vi "Move bimorph.vi"() -> ()   [LabVIEW 2010]
uses:
  <vilib>/express/express analysis/Spectral/XNode/ExpressSpectralMeasurementsBlockNode.xnode
  <vilib>/DAQmx/read.llb/DAQmx Read (Analog 2D DBL NChan NSamp).vi
  <vilib>/daqmx/miscellaneous.llb/DAQmx Fill In Error Info.vi
  <vilib>/express/express analysis/Spectral/Block/exnSpectralBlock spectral measurements peak poly.vi
  <vilib>/express/express analysis/Spectral/Block/exnSpectralBlock spectral measurements peak array WFM.vi
panel:
  out "Amplitude 2 (microns)":sgl=3.0 format="%.4f"
  in  "Load config file":bool
  out "Config file path":path
  in  "Save config file":bool
  in  "Axis":T1(radio)=enum."Radio Selection 3"
  in  "Bimorph scaling factor (?/V)":dbl=1.0
  out "FFT":cluster{"f0":dbl, "df":dbl, "magnitude":dbl[]}[](graph)
  out "Period (s)":dbl
  in  "Timing":T2={"Delay 1 (s)"=10.0, "Duration (s)"=10.0, "Delay 2 (s)"=10.0} {"Delay 2 (s)" step=0.5 format="%.1g"; "Duration (s)" step=0.5 format="%.1g"; "Delay 1 (s)" step=0.5 format="%.1g"}
  out "Coordinates":T3 {"Zcoordinate" format="%.4f"; "Ycoordinate" format="%.4f"; "Xcoordinate" format="%.4f"}
  out "Coordinates (microns)":T4={"Xcoordinate (microns)"=8589, "Ycoordinate (microns)"=6028, "Zcoordinate (microns)"=4319}
  out "Error":bool
  in  "Get start position":bool
  in  "Amplitude 0 (microns)":dbl format="%.4g"
  in  "Shell?":bool
  out "Amplitude index":i32=1
  out "File path":path caption="Saved file path"
  in  "Comments":string
  in  "Save?":bool=TRUE
  in  "stop":bool
  in  "Amplitudes":T5={"# of amplitudes"=1, "Amplitude type?"=0, "Amplitude 1 (microns)"=3.0, "Step size (microns)"=0.0, "Amplitude array (microns)"=[]} {"Amplitude array (microns)" format="%.4g"; "Step size (microns)" step=0.0625 format="%.4f"; "Amplitude 1 (microns)" format="%.4f"; "Amplitude type?" items=["Linear", "Array"]}
  in  "Sample rate (Hz)":dbl=2000.0 format="%.2f"
  out "WAITING?":bool
  in  "CONTINUE":bool
  in  "Switch":u8(slide) step=1 scale=0.0..2.0
  out "Bimorph voltage":cluster{dbl, dbl, "data":dbl[]}(graph)
  in  "AI max value":dbl=10.0 caption="Input Maximum Value" format="%0.2f"
  in  "AI min value":dbl=-10.0 caption="Input Minimum Value" format="%0.2f"
  in  "AI channels":tag="Dev2/ai0" caption="Input Physical Channel"
  # "Channel Parameters"
  # "STOP VI"
  # "IDLE"
  # "RUN"
  # "ai0: Bimorph signal from amplifier"
  # "ENTER BEFORE RUN."
  # "DECIDE BEFORE RUN."
  # "Log file key:\nFile name\nComments\nSample rate (Hz)\nDelay 1 (s)\nDuration (s)\nDelay 2 (s)\nX coordinate (microns)\nY coordinate (microns)\nZ coordinate (microns)\nBimorph scaling factor\nAmplitude 0 (microns)\n# of amplitudes\nAmplitude type (0=linear, 1=array)\nAmplitude 1 (microns)\nStep size (microns)\nSize of amplitude array\nAmpiltude array (microns)"
  # "Instructions:\n1. Run vi.\n2. In IDLE mode, specify the sample rate, the timing parameters, the bimorph scaling factor, and comments.\n3. Choose which axis to control, then get the start position (the baseline of the pulse), amplitude 0.\n4. Specify the amplitude parameters. Note that all amplitudes are absolute, not relative.\n5. Run the Shell if needed, and decide if you want to save.\n6. Click RUN.\n\nNotes:\n-The communication with the Sutter manipulator sometimes has errors. Try to visually confirm on the \nROE that the commanded move is what you want.\n-When setting the timing parameters, make sure to account for the time it takes for the manipulator to\nmove.\n-The minimum step size is 62.5 nm.\n\n-"
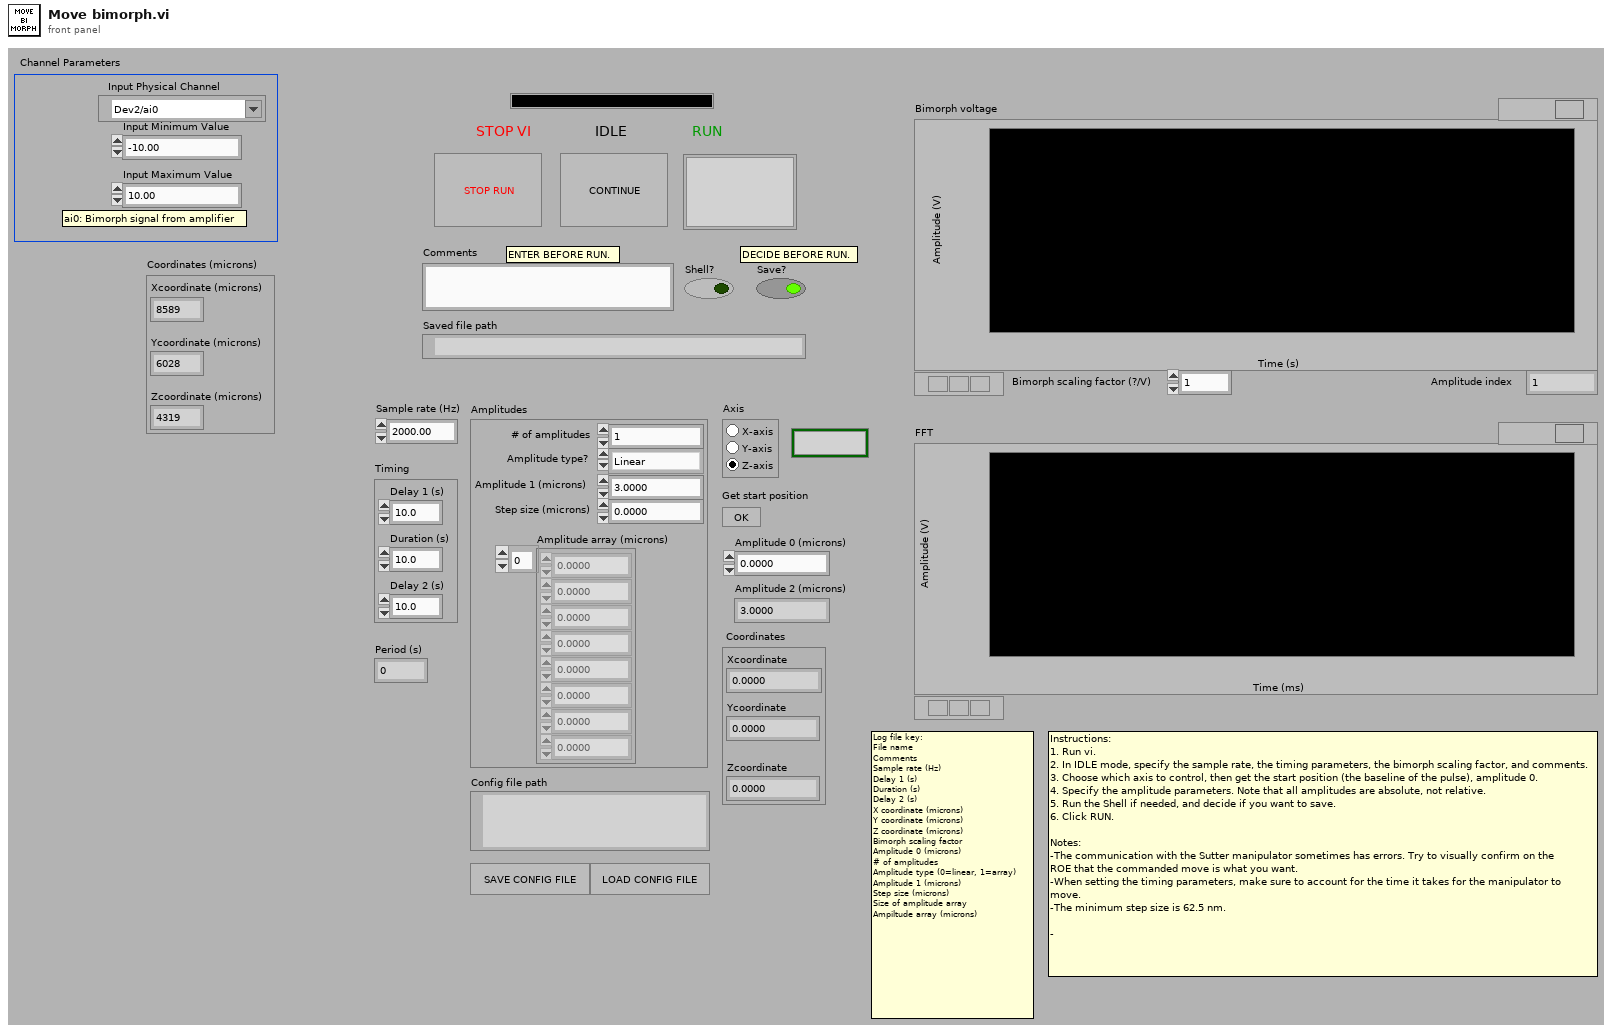
[diagram p1: front panel]
types:
  T1 = enum32{"Radio Selection 1", "Radio Selection 2", "Radio Selection 3"}
  T2 = cluster{"Delay 1 (s)":dbl, "Duration (s)":dbl, "Delay 2 (s)":dbl}
  T3 = cluster{"Xcoordinate ":dbl, "Ycoordinate":dbl, "Zcoordinate":dbl}
  T4 = cluster{"Xcoordinate (microns)":i32, "Ycoordinate (microns)":i32, "Zcoordinate (microns)":i32}
  T5 = cluster{"# of amplitudes":i32, "Amplitude type?":u16, "Amplitude 1 (microns)":sgl, "Step size (microns)":sgl, "Amplitude array (microns)":dbl[]}
  T6 = cluster{"name":string, "type desc":i16[], "flat data":string}[]
  T7 = cluster{"averaging mode":u16, "weighting mode":u16, "number of averages":u32}
  T8 = cluster{"dB On (F)":bool, "unwrap phase (F)":bool, "convert to degree (F)":bool}
  T9 = cluster{"Xcoordinate (not rounded)":dbl, "Ycoordinate (not rounded)":dbl, "Zcoordinate (not rounded)":dbl}
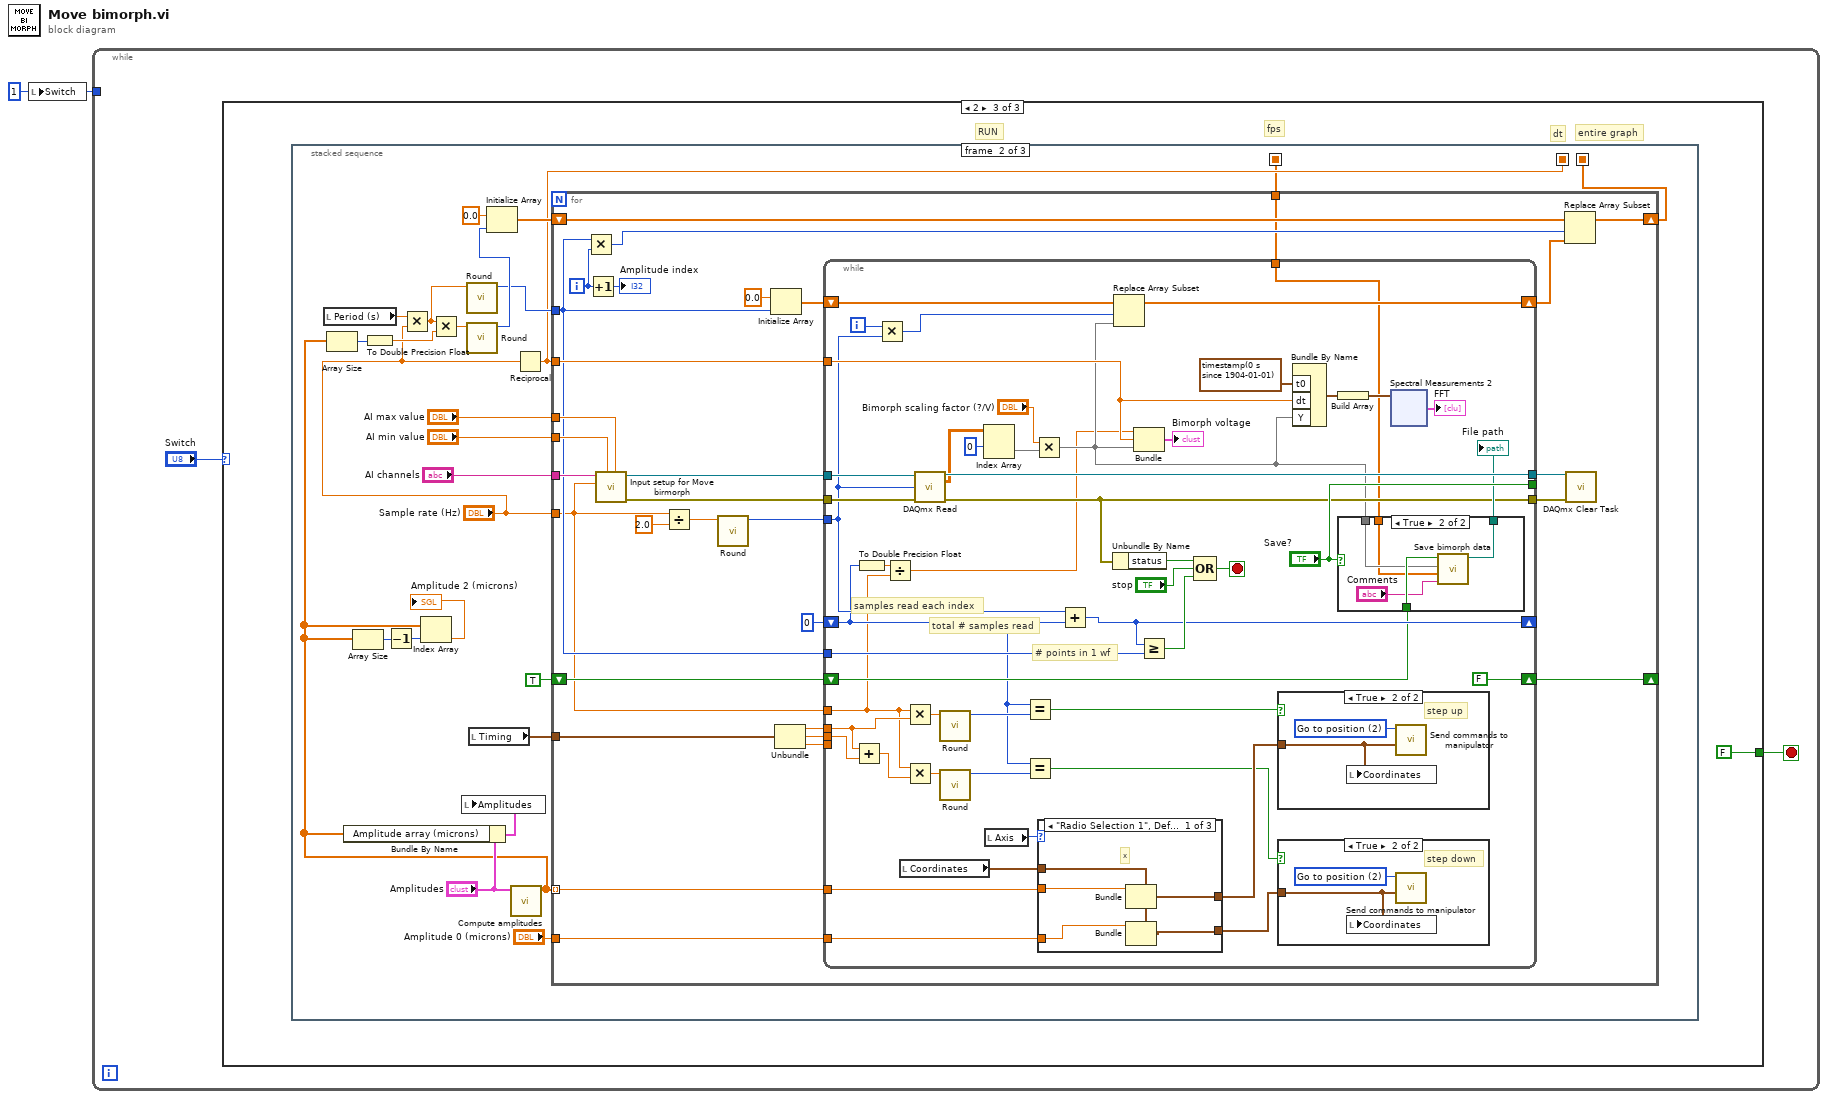
[diagram p0: block diagram]
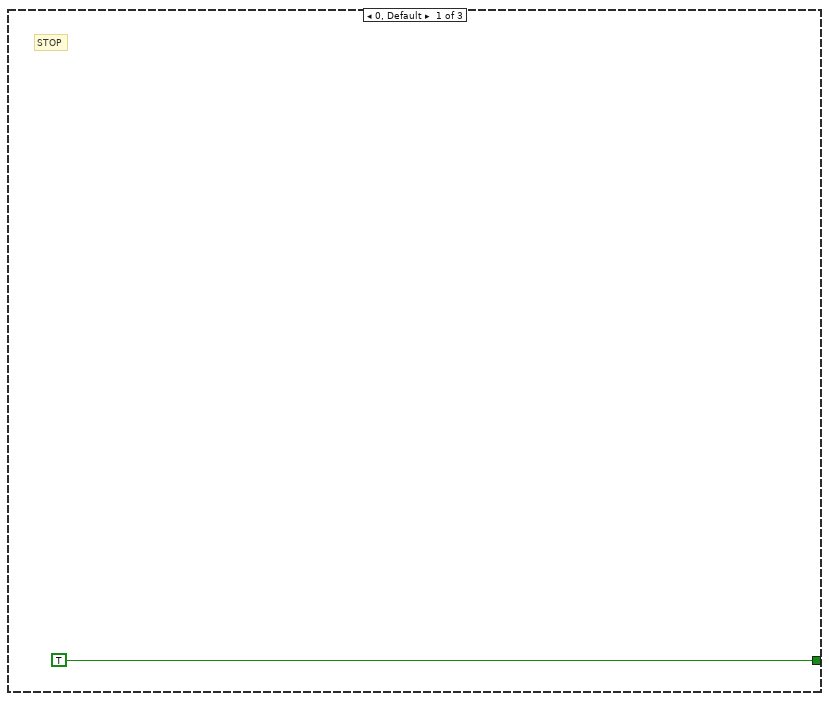
[diagram p2: hidden frame]
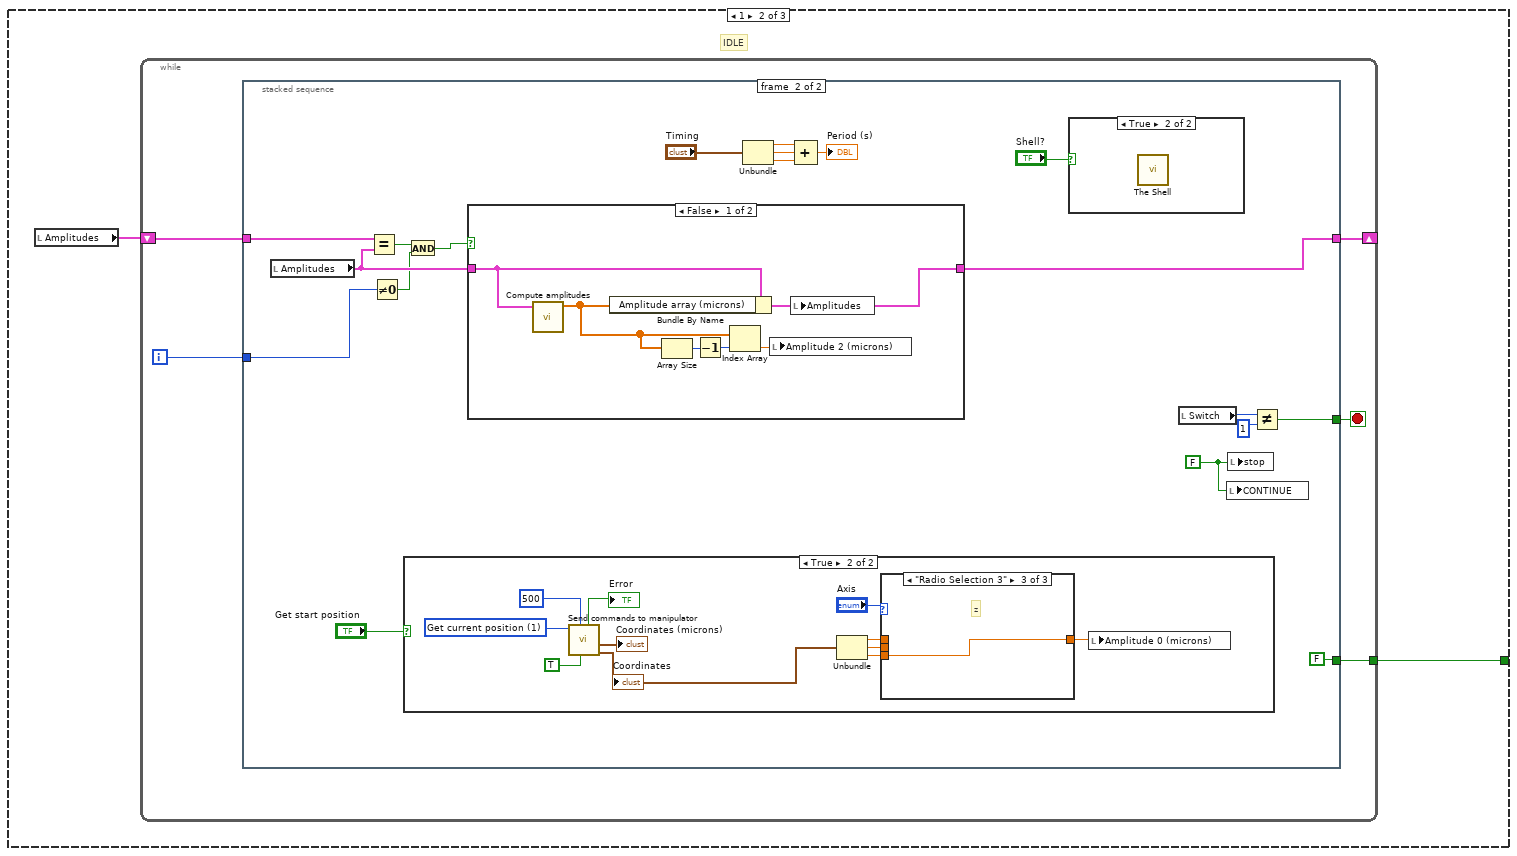
[diagram p3: hidden frame]
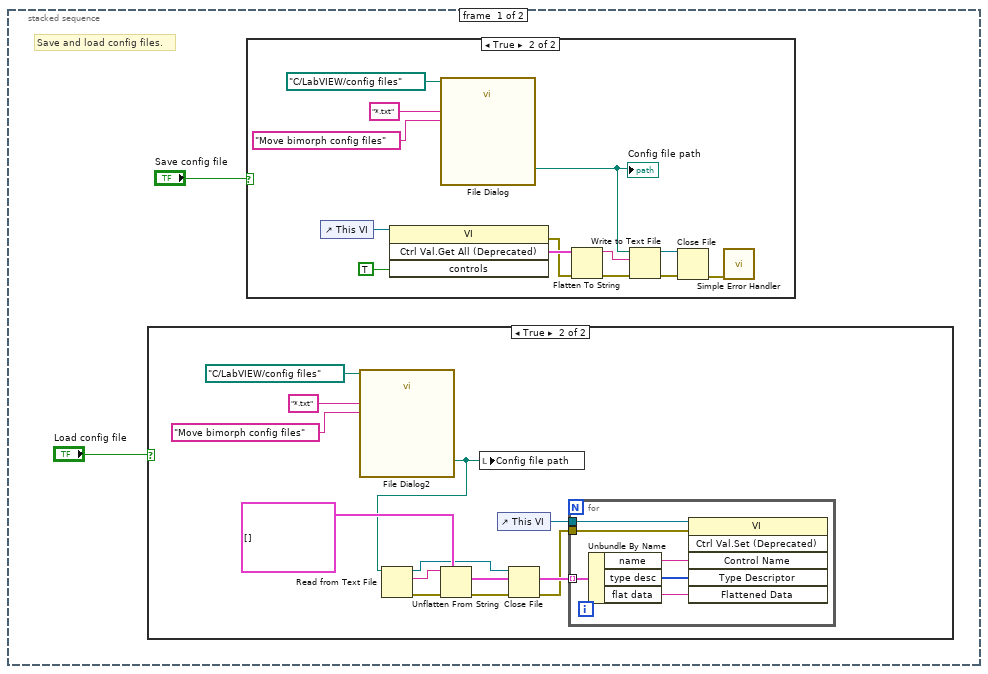
[diagram p4: hidden frame]
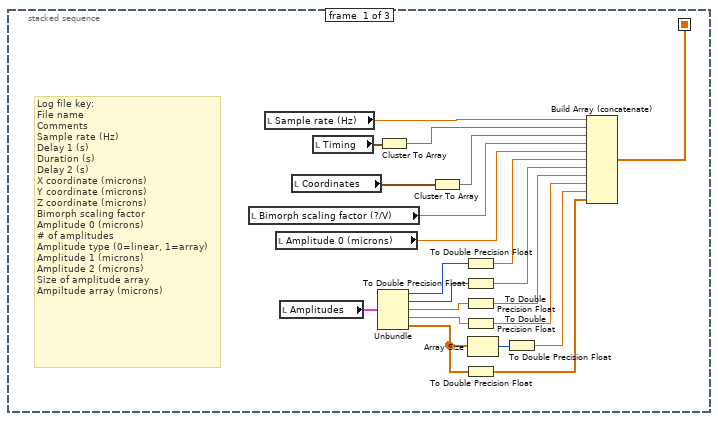
[diagram p12: hidden frame]
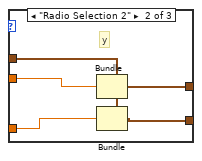
[diagram p14: hidden frame]
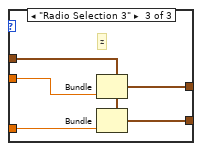
[diagram p15: hidden frame]
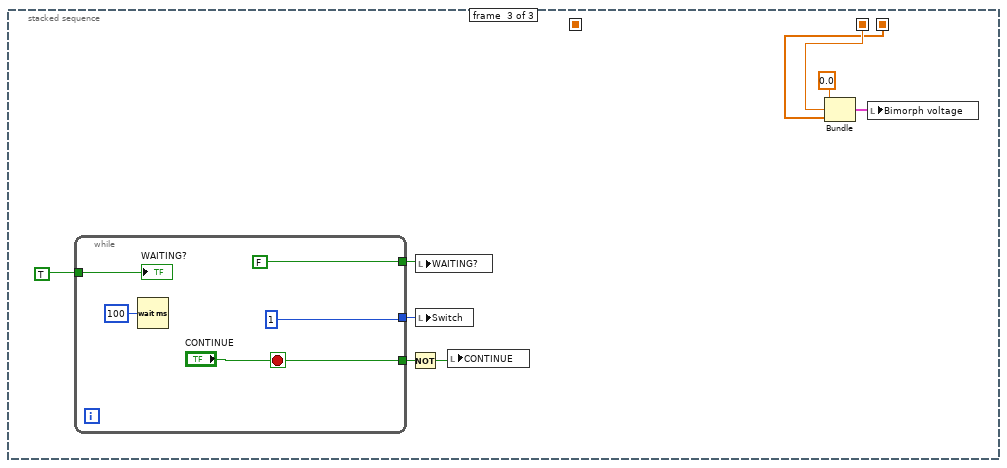
[diagram p18: hidden frame]
diagram:
  w1 = u8 1 ("Switch")
  n1 = local write "Switch"(w1) -> ()
  n2 = while {
    tunnel: w1 -> [_]
    stop <- w2 stop-if-true
    n3 = case shown="2" "Switch" {
      tunnel: [TRUE w6 FALSE] -> w2
      frame 0, Default {
        # "STOP"
      }
      frame 1 {
        # "IDLE"
        n4 = local read "Amplitudes"() -> (w5:T5)
        n5 = while {
          tunnel: [w9] -> w6
          shift-right: [w7] -> _
          shift-left: w5 -> [w8]
          i -> [w11]
          stop <- w10 stop-if-true
          n6 = stacked-sequence {
            tunnel: w11 -> [_ w47]
            tunnel: [_ w59] -> w10
            tunnel: [_ FALSE] -> w9
            tunnel: w8 -> [_ w51]
            tunnel: [_ w49] -> w7
            frame #0 {
              # "Save and load config files."
              n7 = case shown="True" "Load config file" {
                frame False {
                }
                frame True {
                  n8 = call "File Dialog2"("start path"=path "C:/LabVIEW/config files", "pattern (all files)"="*.txt", "pattern label"="Move bimorph config files") -> ("selected path"=w15:path)  [unwired: 9 in, 3 out]
                  n9 = Read from Text File(file (use dialog)=w15) -> (refnum out=w20:refnum<file>, text=w22:string, error out=w21:errorcluster)  [unwired: 1 in, 3 out]
                  n10 = Unflatten From String(type=T6 [] ("Control Value:Get All [Flattened]"), binary string=w22, error in (no error)=w21) -> (value=w24:T6, error out=w19:errorcluster)  [unwired: 3 out]
                  n11 = local write "Config file path"(w15) -> ()
                  n12 = control-ref of="This VI"() -> (w25:refnum<vi>)
                  n13 = Close File(refnum=w20, error in=w19) -> (error out=w14:errorcluster)  [unwired: 1 out]
                  n14 = for {
                    tunnel: w25 -> [w31]
                    tunnel: w24 -> [w30] mode=indexing
                    tunnel: w14 -> [w26]
                    n15 = Unbundle By Name(w30) -> ("name"=w29:string, "type desc"=w28:i16[], "flat data"=w27:string)
                    n16 = invoke class="VI" method="Ctrl Val.Set (Deprecated)"(reference=w31, error in=w26, "Control Name"=w29, "Type Descriptor"=w28, "Flattened Data"=w27) -> ()  [unwired: 1 in, 6 out]
                  }
                }
              }
              n17 = case shown="True" "Save config file" {
                frame False {
                }
                frame True {
                  n18 = control-ref of="This VI"() -> (w40:refnum<vi>)
                  n19 = invoke class="VI" method="Ctrl Val.Get All (Deprecated)"(reference=w40, "controls"=TRUE ("Controls")) -> (error out=w42:errorcluster, "Get All Control Values"=w44:T6)  [unwired: 2 in, 2 out]
                  n20 = call "File Dialog"("start path"=path "C:/LabVIEW/config files", "pattern (all files)"="*.txt", "pattern label"="Move bimorph config files") -> ("selected path"=w32:path)  [unwired: 9 in, 3 out]
                  "Config file path" <- w32
                  n21 = Flatten To String(anything=w44, error in (no error)=w42) -> (data string=w43:string, error out=w41:errorcluster)  [unwired: 3 out]
                  n22 = Write to Text File(file (use dialog)=w32, text=w43, error in=w41) -> (refnum out=w37:refnum<file>, error out=w36:errorcluster)  [unwired: 2 out]
                  n23 = Close File(refnum=w37, error in=w36) -> (error out=w38:errorcluster)  [unwired: 1 out]
                  n24 = call <vilib>:"Simple Error Handler.vi"("error in (no error)"=w38) -> ()  [unwired: 1 in, 8 out]
                }
              }
            }
            frame #1 {
              w63 = FALSE
              n25 = local read "Amplitudes"() -> (w50:T5)
              n26 = Equal?(x=w51, y=w50) -> (x = y?=w48:bool)
              n27 = Not Equal To 0?(x=w47) -> (x != 0?=w46:bool)
              n28 = case shown="True" "Get start position" {
                frame False {
                }
                frame True {
                  w81 = u16 1 items=["Change manipulator", "Get current position", "Go to position", "Home", "Work", "Center", "Interrupt move"] ("Command")
                  n29 = call "Send commands to manipulator.vi"("read"=TRUE, "delay before read (ms)"=u32 500, "Command"=w81) -> ("Coordinates (not rounded)"=w77:T9, "Coordinates (microns)"=→"Coordinates (microns)":T4, "Error"=→"Error":bool)  [unwired: 4 in, 2 out]
                  "Coordinates" <- w77
                  n30 = Unbundle(w77) -> ("Xcoordinate (not rounded)"=w76:dbl, "Ycoordinate (not rounded)"=w75:dbl, "Zcoordinate (not rounded)"=w74:dbl)
                  n31 = case shown="\"Radio Selection 3\"" "Axis" {
                    tunnel: w76 -> [w82 _ _]
                    tunnel: w75 -> [_ w83 _]
                    tunnel: w74 -> [_ _ w84]
                    tunnel: [w82 w83 w84] -> w73
                    frame "Radio Selection 1", Default {
                      # "x"
                    }
                    frame "Radio Selection 2" {
                      # "y"
                    }
                    frame "Radio Selection 3" {
                      # "z"
                    }
                  }
                  n32 = local write "Amplitude 0 (microns)"(w73) -> ()
                }
              }
              n33 = And(x=w48, y=w46) -> (x .and. y?=w45:bool)
              n34 = case shown="False" w45 {
                tunnel: w50 -> [w69 w70]
                tunnel: [w68 w70] -> w49
                frame False {
                  n35 = call "Compute amplitudes.vi"("Run amplitude bundle"=w69) -> ("Amplitudes"=w65:dbl[])  [unwired: 10 in]
                  n36 = Bundle By Name(cluster=w69, "Amplitude array (microns)"=w65) -> (w68:T5)
                  n37 = Array Size(array=w65) -> (size(s)=w67:i32)
                  n38 = Decrement(x=w67) -> (x-1=w66:i32)
                  n39 = Index Array(array=w65, index=w66) -> (element=w64:dbl)
                  n40 = local write "Amplitude 2 (microns)"(w64) -> ()
                  n41 = local write "Amplitudes"(w68) -> ()
                }
                frame True {
                }
              }
              n42 = Unbundle("Timing") -> ("Delay 1 (s)"=w55:dbl, "Duration (s)"=w54:dbl, "Delay 2 (s)"=w53:dbl)
              n43 = Compound Arithmetic op=ADD(w55, w54, w53) -> (→"Period (s)":dbl)
              n44 = case shown="True" "Shell?" {
                frame False {
                }
                frame True {
                  n45 = call "The Shell.vi"() -> ()  [unwired: 1 in]
                }
              }
              n46 = local read "Switch"() -> (w61:u8)
              n47 = local write "CONTINUE"(w63) -> ()
              n48 = local write "stop"(w63) -> ()
              n49 = Not Equal?(x=w61, y=u8 1) -> (x != y?=w59:bool)
            }
          }
        }
      }
      frame 2 {
        # "entire graph"
        # "dt"
        # "fps"
        # "RUN"
        n50 = stacked-sequence {
          seq-local: [_ w128 _] -> [_ _ w247]
          seq-local: [_ w114 _] -> [_ _ w248]
          seq-local: [w86 _ _] -> [_ w113 _]
          frame #0 {
            # "Log file key:\nFile name\nComments\nSample rate (Hz)\nDelay 1 (s)\nDuration (s)\nDelay 2 (s)\nX coordinate (microns)\nY coordinate (microns)\nZ coordinate (microns)\nBimorph scaling factor\nAmplitude 0 (microns)\n# of amplitudes\nAmplitude type (0=linear, 1=array)\nAmplitude 1 (microns)\nAmplitude 2 (microns)\nSize of amplitude array\nAmpiltude array (microns)"
            n51 = local read "Bimorph scaling factor (?/V)"() -> (w96:dbl)
            n52 = local read "Sample rate (Hz)"() -> (w103:dbl)
            n53 = local read "Amplitude 0 (microns)"() -> (w95:dbl)
            n54 = local read "Amplitudes"() -> (w105:T5)
            n55 = local read "Coordinates"() -> (w104:T3)
            n56 = local read "Timing"() -> (w106:T2)
            n57 = Unbundle(w105) -> ("# of amplitudes"=w101:i32, "Amplitude type?"=w100:u16, "Amplitude 1 (microns)"=w99:sgl, "Step size (microns)"=w98:sgl, "Amplitude array (microns)"=w91:dbl[])
            n58 = Cluster To Array(cluster=w106) -> (array=w102:dbl[])
            n59 = Cluster To Array(cluster=w104) -> (array=w97:dbl[])
            n60 = To Double Precision Float(number=w101) -> (double precision float=w94:dbl)
            n61 = To Double Precision Float(number=w100) -> (double precision float=w93:dbl)
            n62 = To Double Precision Float(number=w99) -> (double precision float=w92:dbl)
            n63 = To Double Precision Float(number=w98) -> (double precision float=w90:dbl)
            n64 = To Double Precision Float(number=w91) -> (double precision float=w87:dbl[])
            n65 = Array Size(array=w91) -> (size(s)=w89:i32)
            n66 = To Double Precision Float(number=w89) -> (double precision float=w88:dbl)
            n67 = Build Array (concatenate)(w103, w102, w97, w96, w95, w94, w93, w92, w90, w88, w87) -> (w86:dbl[])
          }
          frame #1 {
            n68 = local read "Period (s)"() -> (w124:dbl)
            n69 = Multiply(x=w124, y="Sample rate (Hz)") -> (x*y=w118:dbl)
            n70 = call "Round.vi"("Number"=w118) -> ("Rounded number"=w117:i32)  [unwired: 10 in]
            n71 = local read "Timing"() -> (w116:T2)
            n72 = call "Compute amplitudes.vi"("Run amplitude bundle"="Amplitudes") -> ("Amplitudes"=w107:dbl[])  [unwired: 10 in]
            n73 = Array Size(array=w107) -> (size(s)=w123:i32)
            n74 = Bundle By Name(cluster="Amplitudes", "Amplitude array (microns)"=w107) -> (w108:T5)
            n75 = Array Size(array=w107) -> (size(s)=w112:i32)
            n76 = To Double Precision Float(number=w123) -> (double precision float=w122:dbl)
            n77 = Decrement(x=w112) -> (x-1=w111:i32)
            n78 = Index Array(array=w107, index=w111) -> (element=→"Amplitude 2 (microns)":dbl)
            n79 = Multiply(x=w118, y=w122) -> (x*y=w121:dbl)
            n80 = local write "Amplitudes"(w108) -> ()
            n81 = call "Round.vi"("Number"=w121) -> ("Rounded number"=w119:i32)  [unwired: 10 in]
            n82 = Initialize Array(0.0 ("element"), w119) -> (w131:dbl[])
            n83 = Reciprocal(x="Sample rate (Hz)") -> (1/x=w114:dbl)
            n84 = for {
              tunnel: "Sample rate (Hz)" -> [w135]
              shift-right: [w158] -> w128
              shift-left: w131 -> [w146]
              shift-right: [w159] -> _
              shift-left: TRUE -> [w160]
              tunnel: "AI channels" -> [w156]
              tunnel: "AI max value" -> [w155]
              tunnel: "AI min value" -> [w154]
              tunnel: w114 -> [w148]
              tunnel: w117 -> [w140]
              tunnel: w116 -> [w139]
              tunnel: w107 -> [w134] mode=indexing
              tunnel: "Amplitude 0 (microns)" -> [w133]
              tunnel: w113 -> [w132]
              i -> [w142]
              n85 = Multiply(x=w140, y=w142) -> (x*y=w141:i32)
              n86 = Increment(x=w142) -> (x+1=→"Amplitude index":i32)
              n87 = call "Input setup for Move birmorph.vi"("AI max value"=w155, "AI min value"=w154, "Sample rate (Hz)"=w135, "AI channels"=w156) -> ("error out"=w152:errorcluster, "AI task out"=w153:refnum<k21>)  [unwired: 6 in]
              n88 = Divide(x=w135, y=2.0) -> (x/y=w150:dbl)
              n89 = call "Round.vi"("Number"=w150) -> ("Rounded number"=w149:i32)  [unwired: 10 in]
              n90 = Initialize Array(0.0 ("element"), w140) -> (w145:dbl[])
              n91 = Unbundle(w139) -> ("Delay 1 (s)"=w138:dbl, "Duration (s)"=w137:dbl, "Delay 2 (s)"=w136:dbl)
              n92 = while {
                shift-right: [w190] -> w143
                shift-left: w145 -> [w193]
                shift-right: [w204] -> _
                shift-left: 0 -> [w168]
                tunnel: [w205] -> w161
                shift-right: [FALSE] -> w159
                shift-left: w160 -> [w203]
                tunnel: ["Save?"] -> _
                tunnel: w153 -> [w198]
                tunnel: w152 -> [w197]
                tunnel: w149 -> [w186]
                tunnel: w148 -> [w195]
                tunnel: [w187] -> w147
                tunnel: w140 -> [w185]
                tunnel: w138 -> [w174]
                tunnel: w137 -> [w173]
                tunnel: w136 -> [_]
                tunnel: w135 -> [w166]
                tunnel: w134 -> [w178]
                tunnel: w133 -> [w169]
                tunnel: w132 -> [w163]
                i -> [w189]
                stop <- w209 stop-if-true
                # "samples read each index"
                # "# points in 1 wf"
                # "total # samples read"
                n93 = Add(x=w174, y=w173) -> (x+y=w172:dbl)
                n94 = To Double Precision Float(number=w168) -> (double precision float=w167:dbl)
                n95 = Multiply(x=w189, y=w186) -> (x*y=w188:i32)
                n96 = Divide(x=w167, y=w166) -> (x/y=w165:dbl)
                n97 = local read "Coordinates"() -> (w180:T3)
                n98 = Multiply(x=w166, y=w174) -> (x*y=w183:dbl)
                n99 = Multiply(x=w166, y=w172) -> (x*y=w175:dbl)
                n100 = call-poly <vilib>:"DAQmx Read.vi"("task/channels in"=w198, "number of samples per channel"=w186, "error in"=w197) -> ("task out"=w205:refnum<k21>, "data"=w200:dbl[][], "error out"=w187:errorcluster)  [unwired: 10 in]
                n101 = call "Round.vi"("Number"=w183) -> ("Rounded number"=w182:i32)  [unwired: 10 in]
                n102 = call "Round.vi"("Number"=w175) -> ("Rounded number"=w176:i32)  [unwired: 10 in]
                n103 = Index Array(array=w200, index (row)=0) -> (element=w192:dbl[])  [unwired: 1 in]
                n104 = local read "Axis"() -> (w179:T1)
                n105 = Equal?(x=w168, y=w182) -> (x = y?=w181:bool)
                n106 = Equal?(x=w168, y=w176) -> (x = y?=w171:bool)
                n107 = Multiply(x="Bimorph scaling factor (?/V)", y=w192) -> (x*y=w184:dbl[])
                n108 = case shown="\"Radio Selection 1\", Default" w179 {
                  tunnel: w180 -> [w217 w222 w227]
                  tunnel: [w218 w223 w228] -> w177
                  tunnel: w178 -> [w219 w224 w229]
                  tunnel: [w215 w220 w226] -> w170
                  tunnel: w169 -> [w216 w221 w225]
                  frame "Radio Selection 1", Default {
                    # "x"
                    n109 = Bundle(cluster=w217, "Xcoordinate"=w219) -> (w218:T3)  [unwired: 2 in]
                    n110 = Bundle(cluster=w217, "Xcoordinate"=w216) -> (w215:T3)  [unwired: 2 in]
                  }
                  frame "Radio Selection 2" {
                    # "y"
                    n111 = Bundle(cluster=w222, "Ycoordinate"=w224) -> (w223:T3)  [unwired: 2 in]
                    n112 = Bundle(cluster=w222, "Ycoordinate"=w221) -> (w220:T3)  [unwired: 2 in]
                  }
                  frame "Radio Selection 3" {
                    # "z"
                    n113 = Bundle(cluster=w227, "Zcoordinate"=w229) -> (w228:T3)  [unwired: 2 in]
                    n114 = Bundle(cluster=w227, "Zcoordinate"=w225) -> (w226:T3)  [unwired: 2 in]
                  }
                }
                n115 = Add(x=w186, y=w168) -> (x+y=w204:i32)
                n116 = Unbundle By Name(w187) -> ("status"=w212:bool)
                n117 = Replace Array Subset(array=w193, new element=w184, index=w188) -> (w190:dbl[])
                n118 = Bundle(w165, w195, w184) -> (→"Bimorph voltage":cluster{dbl, dbl, dbl[]})  [unwired: 1 in]
                n119 = Greater Or Equal?(x=w204, y=w185) -> (x >= y?=w210:bool)
                n120 = Compound Arithmetic op=OR(w212, "stop", w210) -> (w209:bool)
                n121 = case shown="True" w181 {
                  tunnel: w177 -> [_ w230]
                  frame False {
                  }
                  frame True {
                    w231 = u16 2 items=["Change manipulator", "Get current position", "Go to position", "Home", "Work", "Center", "Interrupt move"] ("Command")
                    # "step up"
                    n122 = local write "Coordinates"(w230) -> ()
                    n123 = call "Send commands to manipulator.vi"("Commands (microns)"=w230, "Command"=w231) -> ()  [unwired: 5 in, 5 out]
                  }
                }
                n124 = case shown="True" w171 {
                  tunnel: w170 -> [_ w213]
                  frame False {
                  }
                  frame True {
                    w214 = u16 2 items=["Change manipulator", "Get current position", "Go to position", "Home", "Work", "Center", "Interrupt move"] ("Command")
                    # "step down"
                    n125 = local write "Coordinates"(w213) -> ()
                    n126 = call "Send commands to manipulator.vi"("Commands (microns)"=w213, "Command"=w214) -> ()  [unwired: 5 in, 5 out]
                  }
                }
                n127 = Bundle By Name("t0"=timestamp(0 s since 1904-01-01), "dt"=w195, "Y"=w184) -> (w207:waveform(dbl))  [unwired: 1 in]
                n128 = Build Array(w207) -> (w206:waveform(dbl)[])
                n129 = case shown="True" "Save?" {
                  tunnel: w203 -> [_ w235]
                  tunnel: w184 -> [_ w234]
                  tunnel: [_ w236] -> w199
                  tunnel: w163 -> [_ w232]
                  frame False {
                  }
                  frame True {
                    n130 = call "Save bimorph data.vi"("Comments"="Comments", "Front panel settings"=w232, "Data"=w234, "New file?"=w235) -> ("File path"=w236:path)  [unwired: 7 in]
                  }
                }
                "File path" <- w199
                n131 = xnode ("Spectral Measurements 2")("Signals"=w206) -> ("FFT - (Peak)"=→"FFT":cluster{"f0":dbl, "df":dbl, "magnitude":dbl[]}[])  [unwired: 1 in, 2 out]
              }
              n132 = Replace Array Subset(array=w146, new element=w143, index=w141) -> (w158:dbl[])
              n133 = call <vilib>:"DAQmx Clear Task.vi"("task in"=w161, "error in"=w147) -> ()  [unwired: 13 in, 1 out]
            }
          }
          frame #2 {
            n134 = while {
              tunnel: [u8 1 ("Switch")] -> w255
              tunnel: ["CONTINUE"] -> w254
              tunnel: TRUE ("WAITING?") -> [w258]
              tunnel: [FALSE ("WAITING?")] -> w251
              stop <- "CONTINUE" stop-if-true
              n135 = Wait (ms)(milliseconds to wait=u32 100) -> ()  [unwired: 1 out]
              "WAITING?" <- w258
            }
            n136 = Not(x=w254) -> (.not. x?=w253:bool)
            n137 = local write "WAITING?"(w251) -> ()
            n138 = local write "Switch"(w255) -> ()
            n139 = local write "CONTINUE"(w253) -> ()
            n140 = Bundle("milliseconds to wait"=0.0, w248, w247) -> (w249:cluster{"milliseconds to wait":dbl, dbl, dbl[]})  [unwired: 1 in]
            n141 = local write "Bimorph voltage"(w249) -> ()
          }
        }
      }
    }
  }
